vi "TF_StrainGauge2Force.vi"(2 "Strain Gauge Value [V]":dbl) -> (5 "Force [N]":dbl)   [LabVIEW 2015]
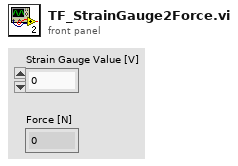
[diagram p1: front panel]
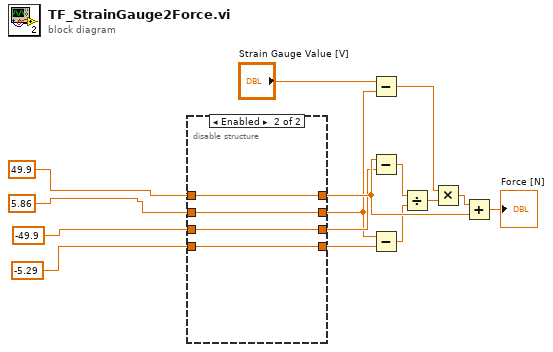
[diagram p0: block diagram]
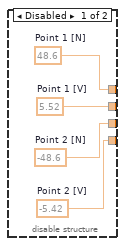
[diagram p2: hidden frame]
diagram:
  n1 = disable-structure shown="Enabled" {
    disable-tunnel: [w19 w23] -> w11
    disable-tunnel: [w18 w21] -> w10
    disable-tunnel: [w17 w22] -> w1
    disable-tunnel: [w16 w20] -> w6
    disable-tunnel: 49.9 -> [_ w23]
    disable-tunnel: 5.86 -> [_ w22]
    disable-tunnel: -49.9 -> [_ w21]
    disable-tunnel: -5.29 -> [_ w20]
    frame Disabled {
      w19 = 48.6  # Point 1 [N]
      w17 = 5.52  # Point 1 [V]
      w18 = -48.6  # Point 2 [N]
      w16 = -5.42  # Point 2 [V]
    }
    frame Enabled {
    }
  }
  n2 = Subtract(x="Strain Gauge Value [V]", y=w1) -> (x-y=w13:dbl)
  n3 = Subtract(x=w11, y=w10) -> (x-y=w9:dbl)
  n4 = Subtract(x=w1, y=w6) -> (x-y=w7:dbl)
  n5 = Divide(x=w9, y=w7) -> (x/y=w8:dbl)
  n6 = Multiply(x=w13, y=w8) -> (x*y=w12:dbl)
  n7 = Add(x=w12, y=w11) -> (x+y=→"Force [N]":dbl)
